vi "Update Course Stage.vi"(8 "Course Stage":i8, 11 "Event":T1) -> (0 "New Course Stage":i8)   [LabVIEW 2016]
uses:
  Event.ctl
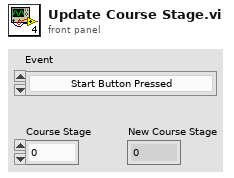
[diagram p1: front panel]
types:
  T1 = typedef "Event.ctl" = enum16{"Start Button Pressed", "Black & Yellow Tape Touched", "Black & Yellow Tape Passed", "Green Tape Crossed", "Red Tape Touched", "Rough Terrain Touched", "Black Tape Crossed", "Tape Edge Too Close", "Wall Too Close", "Rough Terrain Passed", "Ramp Passed", "Stop Button Pressed", "Recentered", "End Zone Wait Timed Out"}
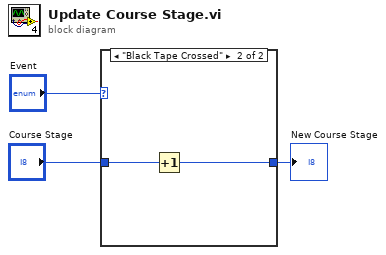
[diagram p0: block diagram]
diagram:
  n1 = case shown="\"Black Tape Crossed\"" "Event" {
    tunnel: "Course Stage" -> [w4 w6]
    tunnel: [w4 w5] -> w1
    frame Default {
    }
    frame "Black Tape Crossed" {
      n2 = Increment(x=w6) -> (x+1=w5:i8)
    }
  }
  "New Course Stage" <- w1
